vi "Event New Child.vi"(8 "error in (no error)":errorcluster, 11 "[V] Tester Parent in":refnum<class "[V] Tester Parent.lvclass">) -> (0 "error out":errorcluster, 3 "[V] Tester Parent out":refnum<class "[V] Tester Parent.lvclass">)   [LabVIEW 2020, in "[V] Tester Parent.lvlib" / "[V] Tester Parent.lvclass"]
uses:
  [V] Tester Parent.lvclass
  D:/iCloudDrive/LabVIEW Tools/LabVIEW-Panel/[MDI] Parent/[MDI] Parent/[MDI] Parent.lvclass
  C:/Program Files (x86)/National Instruments/LabVIEW 2020/vi.lib/ActorFramework/Actor/Actor.lvclass
  [MDI] Parent/[MDI] Parent/[MDI] Parent.lvclass/[MDI] Parent.ctl
  [V] Tester Child/[V] Tester Child/[V] Tester Child.lvclass
  D:/iCloudDrive/LabVIEW Tools/LabVIEW-Panel/[MDI] Child/[MDI] Child/[MDI] Child.lvclass
  [MDI] Child/[MDI] Child/[MDI] Child.lvclass/[MDI] Child.ctl
  [V] Tester Parent.lvclass/[V] Tester Parent.ctl
  [MDI] Parent/[MDI] Parent/Accessor/Read Parent.vi
  [MDI] Child/[MDI] Child/Accessor/Write parent.vi
  [MDI] Child/[MDI] Child/Accessor/Write Child Name.vi
  System.Windows.Forms
  <vilib>/ActorFramework/Actor/Actor.lvclass
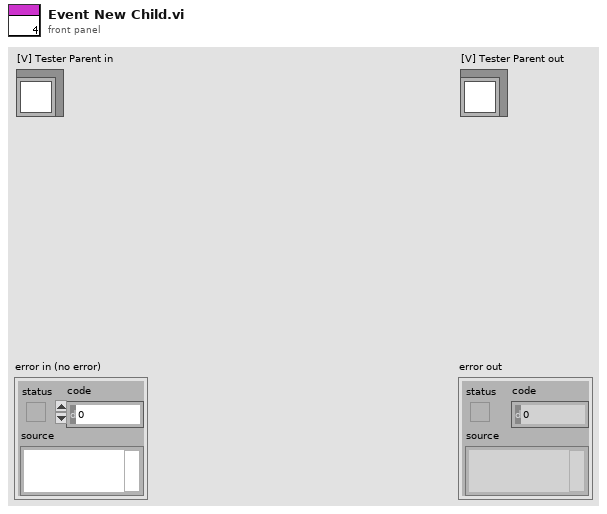
[diagram p1: front panel]
types:
  T1 = map{string, refnum<class "Message Enqueuer.lvclass">}
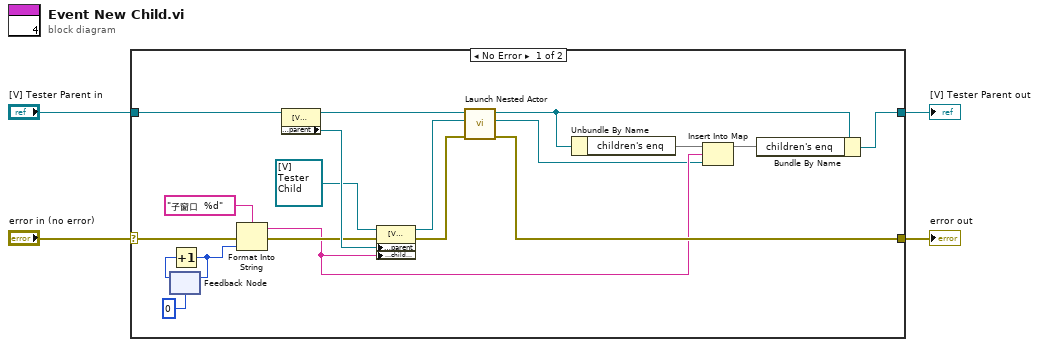
[diagram p0: block diagram]
diagram:
  n1 = case shown="No Error" "error in (no error)" {
    selector: "error in (no error)" -> [w16 w25]
    tunnel: [w17 w25] -> w3
    tunnel: [w6 w24] -> w1
    tunnel: "[V] Tester Parent in" -> [w22 w24]
    frame No Error {
      n2 = feedback #1(0) -> (w12:i32)
      n3 = Increment(x=w12) -> (x+1=w11:i32)
      n4 = feedback-in #1(w11) -> ()
      n5 = Format Into String(format string="子窗口  %d", error in=w16, w11) -> (resulting string=w7:string, error out=w15:errorcluster)  [unwired: 1 in]
      n6 = property class="[V] Tester Parent.lvclass"(reference=w22) -> (reference out=w20:refnum<class "[V] Tester Parent.lvclass">, "Accessor:parent"=w23:refnum<k24>)  [unwired: 1 in, 1 out]
      n7 = property class="[V] Tester Child.lvclass"(reference=refnum<class "[V] Tester Child.lvclass"> refnum ("[V] Tester Child.lvlib:[V] Tester Child.lvclass"), error in=w15, "Accessor:parent"=w23, "Accessor:child name"=w7) -> (reference out=w19:refnum<class "[V] Tester Child.lvclass">, error out=w18:errorcluster)
      n8 = call <vilib>:"Launch Nested Actor.vi"("error in (no error)"=w18, "Nested Actor"=w19, "Caller Actor in"=w20) -> ("error out"=w17:errorcluster, "Nested Actor's Enqueuer"=w5:refnum<class "Message Enqueuer.lvclass">, "Caller Actor out"=w10:refnum<class "[V] Tester Parent.lvclass">)  [unwired: 6 in]
      n9 = Unbundle By Name(w10) -> ("children's enq"=w9:T1)
      n10 = Insert Into Map(map in=w9, key=w7, value=w5) -> (map out=w8:T1)  [unwired: 2 out]
      n11 = Bundle By Name(cluster=w10, "children's enq"=w8) -> (w6:refnum<class "[V] Tester Parent.lvclass">)
    }
    frame Error {
    }
  }
  "error out" <- w3
  "[V] Tester Parent out" <- w1
